vi "Poll He Line Valve Control.vi"(8 "error in (no error)":errorcluster, 11 "He Line in":refnum<class "He Line.lvclass">) -> ()   [LabVIEW 2015, in "cRIO-Carbondioxide.lvlib" / "CO2-Actor.lvlib" / "He Line.lvclass"]
uses:
  He Line.lvclass
  He Line.lvclass/He Line.ctl
  <vilib>/ActorFramework/Actor/Actor.lvclass/Actor.ctl
  <vilib>/ActorFramework/Message Enqueuer/Message Enqueuer.lvclass/Message Enqueuer.ctl
  He Line Messages/Set He Line Msg/Set He Line Msg.lvclass/Set He Line Msg.ctl
  <vilib>/ActorFramework/Actor/Read Self Enqueuer.vi
  <vilib>/ActorFramework/Message Enqueuer/Enqueue.vi
  <vilib>/ActorFramework/Message Enqueuer/Init from Existing Queue.vi
  <vilib>/ActorFramework/Message Priority Queue/Priority Enqueue.vi
  <vilib>/ActorFramework/Actor/Actor.lvclass
  <vilib>/ActorFramework/Message Enqueuer/Message Enqueuer.lvclass
  He Line Messages/Set He Line Msg/Set He Line Msg.lvclass
  cRIO-CO2/cRIO-CO2.lvclass
  CO2 Actor/CO2 Actor.lvclass
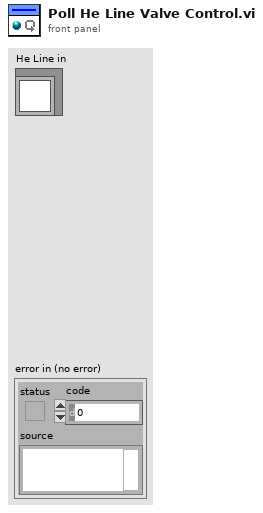
[diagram p1: front panel]
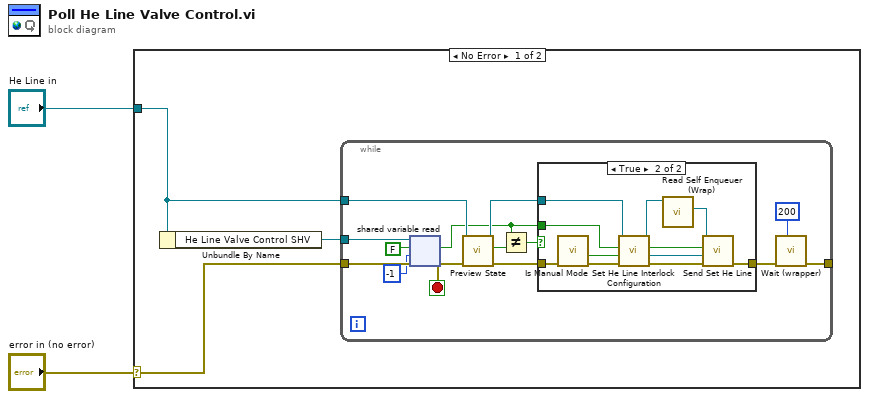
[diagram p0: block diagram]
diagram:
  n1 = case shown="No Error" "error in (no error)" {
    selector: "error in (no error)" -> [w3 _]
    tunnel: "He Line in" -> [w4 _]
    frame No Error {
      n2 = Unbundle By Name(w4) -> ("He Line Valve Control SHV"=w5:refnum<k21>)
      n3 = while {
        tunnel: w5 -> [w19]
        tunnel: w3 -> [w18]
        tunnel: w4 -> [w13]
        tunnel: [w7] -> _
        stop <- w15 stop-if-true
        n4 = shared-variable-read(w19, w18, FALSE, -1 ("timeout ms")) -> (w15:errorcluster, w10:bool)  [unwired: 3 out]
        n5 = call "Preview State.vi"("error in (no error)"=w15, "He Line in"=w13) -> ("error out"=w14:errorcluster, "Is Open?"=w11:bool, "He Line out"=w12:refnum<class "He Line.lvclass">)  [unwired: 7 in]
        n6 = Not Equal?(x=w10, y=w11) -> (x != y?=w9:bool)
        n7 = case shown="True" w9 {
          tunnel: [w20 w30] -> w8
          tunnel: w14 -> [w20 w29]
          tunnel: w12 -> [_ w26]
          tunnel: w10 -> [_ w24]
          frame False {
          }
          frame True {
            n8 = call "Is Manual Mode.vi"("error in (no error)"=w29) -> ("error out"=w28:errorcluster, "Manual Mode?"=w22:bool)  [unwired: 9 in]
            n9 = call "Set He Line Interlock Configuration.vi"("error in (no error)"=w28, "Manual Mode (False)"=w22, "Open? (False)"=w24, "He Line in"=w26) -> ("error out"=w27:errorcluster, "Interlock Chain"=w21:refnum<class "Interlock Chain.lvclass">, "Open? (False) 2"=w23:bool, "He Line out"=w25:refnum<class "He Line.lvclass">)  [unwired: 4 in]
            n10 = call "Read Self Enqueuer (Wrap).vi"("CO2 Actor in"=w25) -> ("Actor Framework:Message Enqueuer"=w31:refnum<class "Message Enqueuer.lvclass">)  [unwired: 9 in, 1 out]
            n11 = call "Send Set He Line.vi"("error in (no error)"=w27, "Interlock Chain"=w21, "Open/Close (Close)"=w23, "Message Enqueuer"=w31) -> ("error out"=w30:errorcluster)  [unwired: 6 in, 1 out]
          }
        }
        n12 = call "Wait (wrapper).vi"("milliseconds to wait (200)"=u32 200 ("milliseconds to wait"), "error in (no error)"=w8) -> ("error out"=w7:errorcluster)  [unwired: 9 in]
      }
    }
    frame Error {
    }
  }
